vi "BuildZoomNames.vi"(10 "History":bool, 11 "WaveformGraph in":refnum<vi>) -> (2 "Names":string[](array[string]))   [LabVIEW 2022 SP3]
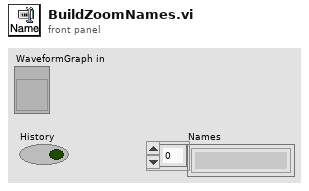
[diagram p1: front panel]
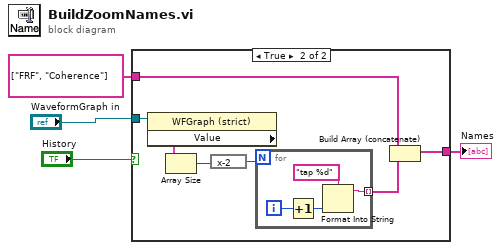
[diagram p0: block diagram]
diagram:
  n1 = case shown="True" "History" {
    tunnel: [w5 w6] -> w2
    tunnel: string[] ["FRF", "Coherence"] ("Names") -> [w5 w8]
    tunnel: "WaveformGraph in" -> [_ w12]
    frame False {
    }
    frame True {
      n2 = property class="WFGraph (strict)"(reference=w12) -> ("Value"=w11:cluster{dbl, "dt":dbl, "Y":dbl[]}[])  [unwired: 1 in, 2 out]
      n3 = Array Size(array=w11) -> (size(s)=w10:i32)
      n4 = expression code="x-2"(w10) -> (w9:i32)
      n5 = for {
        N: w9 -> [_]
        tunnel: [w14] -> w7 mode=indexing
        i -> [w15]
        n6 = Increment(x=w15) -> (x+1=w13:i32)
        n7 = Format Into String(format string="tap %d", w13) -> (resulting string=w14:string)  [unwired: 2 in, 1 out]
      }
      n8 = Build Array (concatenate)(w8, w7) -> (w6:string[])
    }
  }
  "Names" <- w2
